vi "U6 eDO Example.vi"() -> (0 "error out":errorcluster)   [LabVIEW 2021]
panel:
  in  "Address":string="192.168.1.209"
  in  "FirstFound":bool=TRUE
  in  "State":bool
  in  "Channel":i32
  out "Error Message":string
  # "Sets 1 digital output using the UD easy function eDO."
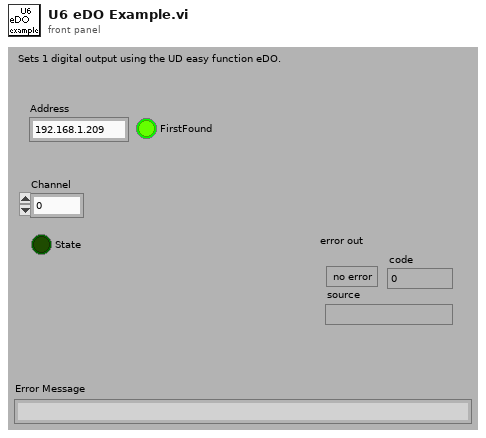
[diagram p1: front panel]
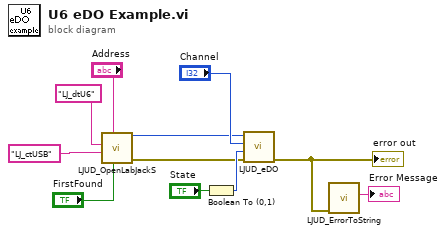
[diagram p0: block diagram]
diagram:
  n1 = call "LJUD_OpenLabJackS.vi"("FirstFound"="FirstFound", "Address"="Address", "ConnectionType"="LJ_ctUSB", "DeviceType"="LJ_dtU6") -> ("error out"=w2:errorcluster, "Handle"=w3:i32)  [unwired: 5 in, 1 out]
  n2 = Boolean To (0,1)(Boolean="State") -> (0, 1=w7:i16)
  n3 = call "LJUD_eDO.vi"("error in"=w2, "State"=w7, "Channel"="Channel", "Handle In"=w3) -> ("error out"=w10:errorcluster)  [unwired: 6 in, 1 out]
  "error out" <- w10
  n4 = call "LJUD_ErrorToString.vi"("error in"=w10) -> ("String"=→"Error Message":string)  [unwired: 10 in]
